vi "1L24_conv_fahreneit_degreC.vi"(1 "Deg F":dbl=100.0 format="%.2f") -> (0 "Deg C":dbl format="%.2f")   [LabVIEW 2010, in "lv_01.lvlib"]
doc: "Conversion de degré Fahrenheit en Celsius"
uses:
  lv_01.lvlib
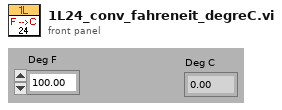
[diagram p1: front panel]
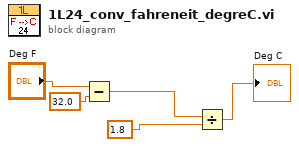
[diagram p0: block diagram]
diagram:
  n1 = Subtract(x="Deg F", y=32.0) -> (x-y=w2:dbl)
  n2 = Divide(x=w2, y=1.8) -> (x/y=→"Deg C":dbl)
